vi "VeriStand Framework Configuration.Create.vi"(8 "error in (no error)":errorcluster, 10 "configuration path":path, 11 "Device Item Ref":T1=18446744073709551615 format="%.0x") -> (0 "error out":errorcluster, 3 "VeriStand Framework Configuration":refnum<class "VeriStand DSF.Framework.Configuration.lvclass">)   [LabVIEW 2017, in "Data Sharing Framework Engine.lvlib" / "VeriStand DSF.Framework.Configuration.lvclass"]
uses:
  VeriStand DSF.Framework.Configuration.lvclass
  DSF Core/Built/Windows/Engine/DSF.Engine.lvlibp/Shared/Classes/Framework/DSF.Shared.Configuration.Framework.lvclass
  <vilib>/NI Veristand/Custom Device API/Custom Device API.lvlib
  VeriStand DSF.Plugin.Configuration.lvclass
  C:/Git/DSF/DSF Core/Built/Windows/Engine/DSF.Engine.lvlibp/Shared/Classes/Framework/DSF.Shared.Configuration.Framework.lvclass
  C:/Git/DSF/DSF Core/Built/Windows/Engine/DSF.Engine.lvlibp/Shared/Classes/Configuration/DSF.Shared.Configuration.lvclass
  VeriStand DSF.Transfer Group.Configuration.lvclass
  VeriStand DSF.Transfer.Configuration.lvclass
  C:/Git/DSF/DSF Core/Built/Windows/Engine/DSF.Engine.lvlibp/Shared/Classes/Plugin/DSF.Shared.Configuration.Plugin.lvclass
  <vilib>/NI Veristand/Custom Device API/Custom Device Item Ref.ctl
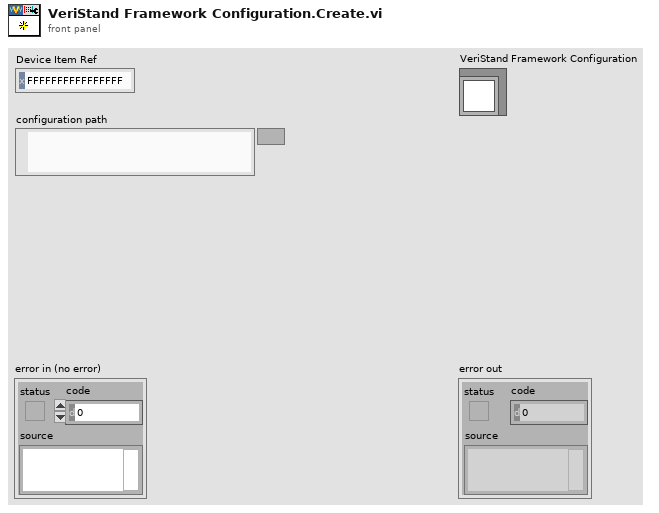
[diagram p1: front panel]
types:
  T1 = typedef "Custom Device API.lvlib/Custom Device Item Ref.ctl" = u64
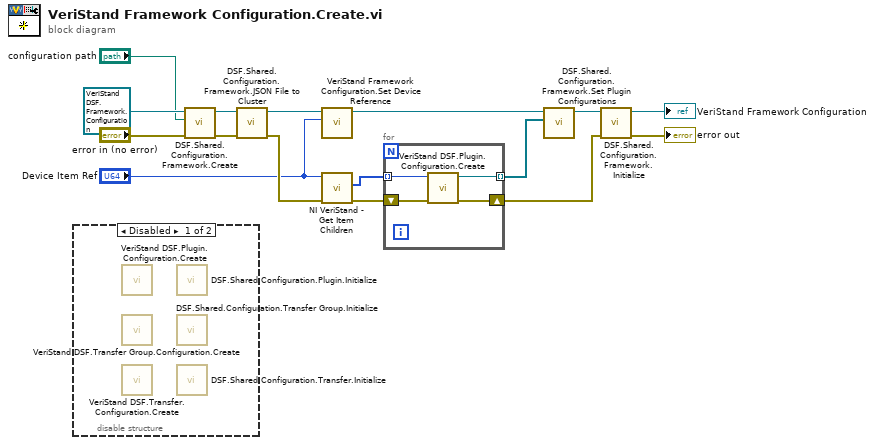
[diagram p0: block diagram]
diagram:
  n1 = disable-structure shown="Disabled" {
    frame Disabled {
      n2 = call "VeriStand DSF.Plugin.Configuration.Create.vi"() -> ()  [unwired: 10 in, 2 out]
      n3 = call "VeriStand DSF.Transfer Group.Configuration.Create.vi"() -> ()  [unwired: 10 in, 2 out]
      n4 = call "VeriStand DSF.Transfer.Configuration.Create.vi"() -> ()  [unwired: 10 in, 2 out]
      n5 = call-dynamic "DSF.Shared.Configuration.Plugin.Initialize.vi"() -> ()  [unwired: 10 in, 2 out]
      n6 = call-dynamic "DSF.Shared.Configuration.Transfer Group.Initialize.vi"() -> ()  [unwired: 10 in, 2 out]
      n7 = call-dynamic "DSF.Shared.Configuration.Transfer.Initialize.vi"() -> ()  [unwired: 10 in, 2 out]
    }
    frame Enabled {
    }
  }
  n8 = call "DSF.Shared.Configuration.Framework.Create.vi"("error in (no error)"="error in (no error)", "configuration path"="configuration path", "Framework Configuration type"=refnum<class "VeriStand DSF.Framework.Configuration.lvclass"> refnum ("VeriStand Framework Configuration in")) -> ("error out"=w9:errorcluster, "Framework Configuration"=w11:refnum<class "VeriStand DSF.Framework.Configuration.lvclass">)  [unwired: 7 in]
  n9 = call "DSF.Shared.Configuration.Framework.JSON File to Cluster.vi"("error in (no error)"=w9, "Framework Configuration in"=w11) -> ("error out"=w7:errorcluster, "Framework Configuration out"=w12:refnum<class "VeriStand DSF.Framework.Configuration.lvclass">)  [unwired: 8 in]
  n10 = call "VeriStand Framework Configuration.Set Device Reference.vi"("Device Item Ref"="Device Item Ref", "VeriStand Framework Configuration in"=w12) -> ("VeriStand Framework Configuration out"=w13:refnum<class "VeriStand DSF.Framework.Configuration.lvclass">)  [unwired: 9 in]
  n11 = call <vilib>:"NI VeriStand - Get Item Children.vi"("error in (no error)"=w7, "Item Ref in"="Device Item Ref") -> ("error out"=w16:errorcluster, "Child Refs"=w15:T1[])  [unwired: 6 in, 2 out]
  n12 = for {
    shift-right: [w19] -> w2
    shift-left: w16 -> [w20]
    tunnel: [w18] -> w14 mode=indexing
    tunnel: w15 -> [w17] mode=indexing
    n13 = call "VeriStand DSF.Plugin.Configuration.Create.vi"("error in (no error)"=w20, "Section Ref"=w17) -> ("error out"=w19:errorcluster, "Plugin Configuration"=w18:refnum<class "VeriStand DSF.Plugin.Configuration.lvclass">)  [unwired: 8 in]
  }
  n14 = call "DSF.Shared.Configuration.Framework.Set Plugin Configurations.vi"("Plugin Configurations"=w14, "Framework Configuration in"=w13) -> ("Framework Configuration out"=w4:refnum<class "VeriStand DSF.Framework.Configuration.lvclass">)  [unwired: 9 in]
  n15 = call-dynamic "DSF.Shared.Configuration.Framework.Initialize.vi"("error in (no error)"=w2, "Framework Configuration in"=w4) -> ("error out"=→"error out":errorcluster, "Framework Configuration out"=→"VeriStand Framework Configuration":refnum<class "VeriStand DSF.Framework.Configuration.lvclass">)  [unwired: 8 in]
